vi "Type Specialization Structure - Lesson 1.vi"() -> ()   [LabVIEW 2023]
doc: "Lesson 1 looks at a simple use of the <b>Type Specialization</b> structure in a malleable VI that ships with LabVIEW."
uses:
  b53de050-1710-450e-af63-8221b42db9ac.vi
  ae176f51-855b-481c-9f50-9a0c565a0305.vi
panel:
  out "array out 2":i32[](array[numeric])
  out "array out 1":i32[](array[numeric])
  # "Overview: This example assumes you are familiar with malleable VIs. If you are not, please begin with the examples\\Malleable VIs\\Basics. This example shows you how to use the Type Specialization structure to increase the flexibility of malleable VIs.\n\nThis first lesson looks at a simple use of the Type Specialization structure in a VIM that ships with LabVIEW.\n\nInstructions: \n1. Open the block diagram of this VI. Review the lessons presented there.\n2. Run the VI to see the results. \n3. Once you have finished reviewing this VI, open the next lesson VI in the Malleable VIs - Type Specialization Structure example project."
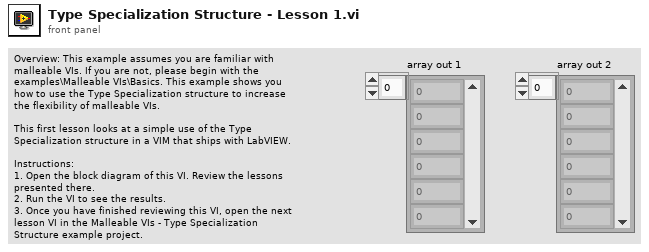
[diagram p1: front panel]
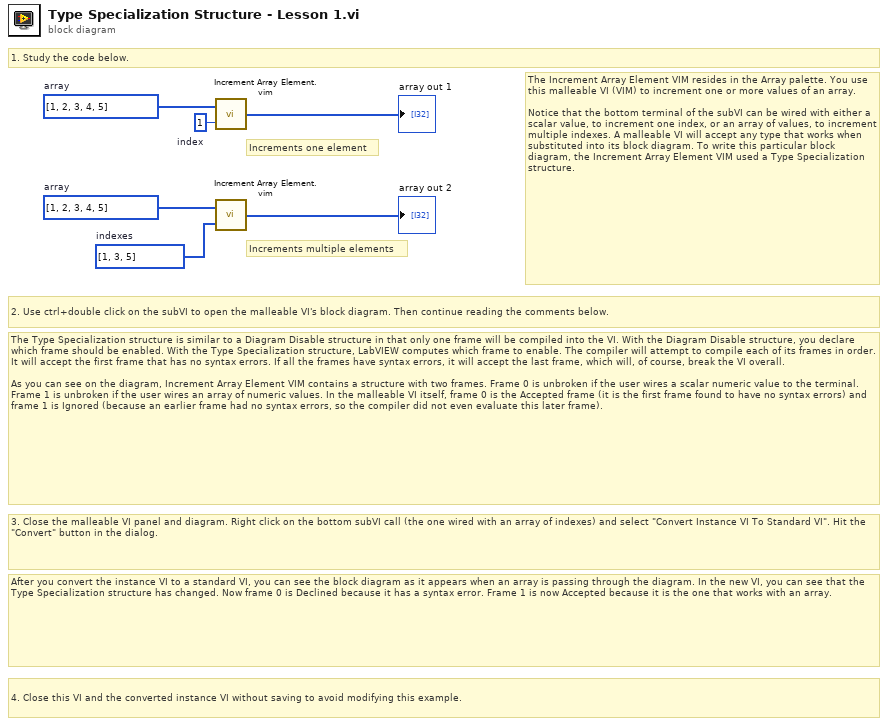
[diagram p0: block diagram]
diagram:
  w2 = i32[] [1, 3, 5]  # indexes
  w3 = i32[] [1, 2, 3, 4, 5]  # array
  w1 = 1  # index
  w6 = i32[] [1, 2, 3, 4, 5]  # array
  # "4. Close this VI and the converted instance VI without saving to avoid modifying this example."
  # "After you convert the instance VI to a standard VI, you can see the block diagram as it appears when an array is passing through the diagram. In the new VI, you can see that the Type Specialization structure has changed. Now frame 0 is Declined because it has a syntax error. Frame 1 is now Accepted because it is the one that works with an array."
  # "3. Close the malleable VI panel and diagram. Right click on the bottom subVI call (the one wired with an array of indexes) and select \"Convert Instance VI To Standard VI\". Hit the \"Convert\" button in the dialog."
  # "The Type Specialization structure is similar to a Diagram Disable structure in that only one frame will be compiled into the VI. With the Diagram Disable structure, you declare which frame should be enabled. With the Type Specialization structure, LabVIEW computes which frame to enable. The compiler will attempt to compile each of its frames in order. It will accept the first frame that has no syntax errors. If all the frames have syntax errors, it will accept the last frame, which will, of course, break the VI overall. \n\nAs you can see on the diagram, Increment Array Element VIM contains a structure with two frames. Frame 0 is unbroken if the user wires a scalar numeric value to the terminal. Frame 1 is unbroken if the user wires an array of numeric values. In the malleable VI itself, frame 0 is the Accepted frame (it is the first frame found to have no syntax errors) and frame 1 is Ignored (because an earlier frame had no syntax errors, so the compiler did not even evaluate this later frame)."
  # "2. Use ctrl+double click on the subVI to open the malleable VI's block diagram. Then continue reading the comments below."
  # "The Increment Array Element VIM resides in the Array palette. You use this malleable VI (VIM) to increment one or more values of an array.\n\nNotice that the bottom terminal of the subVI can be wired with either a scalar value, to increment one index, or an array of values, to increment multiple indexes. A malleable VI will accept any type that works when substituted into its block diagram. To write this particular block diagram, the Increment Array Element VIM used a Type Specialization structure."
  # "Increments multiple elements"
  # "Increments one element"
  # "1. Study the code below."
  n1 = call "Increment Array Element.vim"("index"=w1, "array in"=w6) -> ("array out"=→"array out 1":i32[])
  n2 = call "Increment Array Element.vim"("index"=w2, "array in"=w3) -> ("array out"=→"array out 2":i32[])
